vi "Characters_to_string.vi"(1 "stringIn":string, 2 "Characters to write":string, 3 "Label for characters":string) -> (0 "Output string":string)   [LabVIEW 2020]
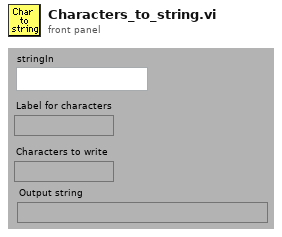
[diagram p1: front panel]
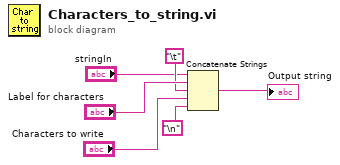
[diagram p0: block diagram]
diagram:
  n1 = Concatenate Strings("stringIn", "Label for characters", "\t", "Characters to write", "\n") -> (→"Output string":string)
